vi "MasterAccelerometerSample6.vi"   [LabVIEW 2016]
uses:
  <vilib>/rvi/Emulation/niFpgaGetClockAttributes.vi
  <vilib>/rvi/Emulation/niFpgaSctlEmulationGetInTimedLoop.vi
  <vilib>/rvi/Emulation/niFpgaEmulationReportErrorSimple.vi
  <vilib>/rvi/eio/common/nirviEmuTemplateMethod_errors.vi
  <vilib>/rvi/Emulation/niFpgaEmulationIsFPGAContextNoSignature.vi
  <vilib>/rvi/DataTransferAndStorage/Container/Common/niFpgaContainerGetUniqueNameForEmu.vi
  <vilib>/rvi/Memory/Memory_Emulation/niFpgaMemoryEmulationCacheClearOnFirstRun.vi
  <vilib>/rvi/Memory/Memory_Emulation/nirvimemoryEmulationManagerCache_MakeExclusive.vi
  <vilib>/rvi/Memory/Memory_Emulation/niFpgaMemoryEmulationValidateCache.vi
  <vilib>/rvi/Memory/Memory_Emulation/nirvimemoryEmulationManagerCache_InsertValue.vi
  <vilib>/Utility/error.llb/Clear Errors.vi
  <vilib>/rvi/Memory/Memory_Emulation/nirvimemoryEmulationManagerCache_ReleaseExclusive.vi
  <vilib>/rvi/Memory/Memory_Emulation/nirvimemoryEmulationManagerCache_GetValue.vi
  <vilib>/rvi/Memory/Memory_Emulation/nirvimemoryEmulationManagerCache_SetValue.vi
  <vilib>/rvi/Emulation/niFpgaProcessEmulError.vi
  <vilib>/rvi/errors/niFpgaSetErrorForExecOnDevCompSimple.vi
  <vilib>/rvi/eio/common/nirviEmuReportErrorAndStop.vi
  <vilib>/rvi/FIFO/Fifo_Resource/nirvififoEmulationSetSize.vi
  <vilib>/rvi/FIFO/Fifo_Resource/nirviFifoEmulationQueueMgr.vi
  <instcachedir>/0/nirviFifoEmulationQueueMgr_E5CAEC123FF24DC58D834DCA3CDAA9B5.lvgen/nirviFifoEmulationQueueMgr_E5CAEC123FF24DC58D834DCA3CDAA9B5_007.vi
  <vilib>/rvi/FIFO/Fifo_Resource/nirvififoEmulationDetermineInputValidOut.vi
  <vilib>/rvi/FIFO/Fifo_Resource/nirvififoEmulationCreateLock.vi
  <vilib>/rvi/FIFO/Fifo_Resource/nirvififoEmulationObtainLock.vi
  <vilib>/rvi/FIFO/Fifo_Resource/nirvififoEmulationReleaseLock.vi
  <vilib>/rvi/occurrence/nirviWaitOnOccurrenceBase.vi
  <vilib>/rvi/errors/nirviReportUnexpectedCaseInternalError.vi
  <vilib>/rvi/errors/nirviReportUnexpectedCaseInternalError (U32).vi
  <instcachedir>/0/nirviFifoEmulationQueueMgr_E5CAEC123FF24DC58D834DCA3CDAA9B5.lvgen/nirviFifoEmulationQueueMgr_E5CAEC123FF24DC58D834DCA3CDAA9B5_005.vi
  <vilib>/rvi/Emulation/niFpgaCriticalErrorInLSC.vi
  <vilib>/eio/EIOMethodNode/EIOMethodNode.xnode
  <vilib>/eio/EIONode/EIONode.xnode
  <vilib>/rvi/DataTransferAndStorage/Container/XNode/niFpgaContainer.xnode
  <vilib>/rvi/DataTransferAndStorage/Register/Emulation/niFpgaRegisterEmulation.vi
  <vilib>/rvi/FIFO/Fifo_Resource/nirvififoEmulationWrite.vi
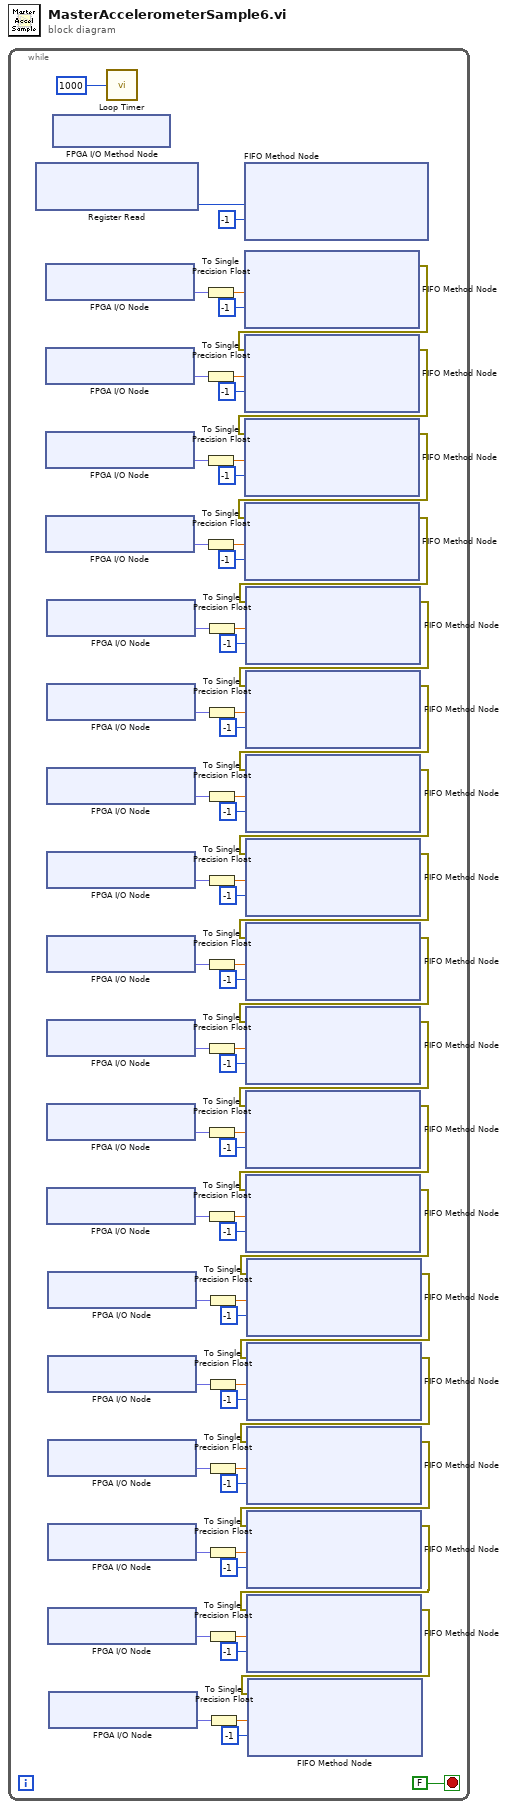
[diagram p0: block diagram]
diagram:
  n1 = while {
    stop <- FALSE stop-if-true
    n2 = xnode ("Register Read")() -> ("Data"=w60:u64)  [unwired: 1 in, 1 out]
    n3 = xnode "FPGA I/O Node"() -> ("Accelerometer1/AI0"=w72:fxp<+/-,24,7>)  [unwired: 1 in, 1 out]
    n4 = xnode "FPGA I/O Node"() -> ("Accelerometer1/AI1"=w67:fxp<+/-,24,7>)  [unwired: 1 in, 1 out]
    n5 = xnode "FPGA I/O Node"() -> ("Accelerometer1/AI2"=w62:fxp<+/-,24,7>)  [unwired: 1 in, 1 out]
    n6 = xnode "FPGA I/O Node"() -> ("Accelerometer2/AI0"=w59:fxp<+/-,24,7>)  [unwired: 1 in, 1 out]
    n7 = xnode "FPGA I/O Node"() -> ("Accelerometer2/AI1"=w42:fxp<+/-,24,7>)  [unwired: 1 in, 1 out]
    n8 = xnode "FPGA I/O Node"() -> ("Accelerometer2/AI2"=w47:fxp<+/-,24,7>)  [unwired: 1 in, 1 out]
    n9 = xnode "FPGA I/O Node"() -> ("Accelerometer3/AI0"=w55:fxp<+/-,24,7>)  [unwired: 1 in, 1 out]
    n10 = xnode "FPGA I/O Node"() -> ("Accelerometer3/AI1"=w50:fxp<+/-,24,7>)  [unwired: 1 in, 1 out]
    n11 = xnode "FPGA I/O Node"() -> ("Accelerometer3/AI2"=w10:fxp<+/-,24,7>)  [unwired: 1 in, 1 out]
    n12 = xnode "FPGA I/O Node"() -> ("Accelerometer4/AI0"=w15:fxp<+/-,24,7>)  [unwired: 1 in, 1 out]
    n13 = xnode "FPGA I/O Node"() -> ("Accelerometer4/AI1"=w23:fxp<+/-,24,7>)  [unwired: 1 in, 1 out]
    n14 = xnode "FPGA I/O Node"() -> ("Accelerometer4/AI2"=w18:fxp<+/-,24,7>)  [unwired: 1 in, 1 out]
    n15 = xnode "FPGA I/O Node"() -> ("Accelerometer5/AI0"=w39:fxp<+/-,24,7>)  [unwired: 1 in, 1 out]
    n16 = xnode "FPGA I/O Node"() -> ("Accelerometer5/AI1"=w34:fxp<+/-,24,7>)  [unwired: 1 in, 1 out]
    n17 = xnode "FPGA I/O Node"() -> ("Accelerometer5/AI2"=w26:fxp<+/-,24,7>)  [unwired: 1 in, 1 out]
    n18 = xnode "FPGA I/O Node"() -> ("Accelerometer6/AI0"=w31:fxp<+/-,24,7>)  [unwired: 1 in, 1 out]
    n19 = xnode "FPGA I/O Node"() -> ("Accelerometer6/AI1"=w8:fxp<+/-,24,7>)  [unwired: 1 in, 1 out]
    n20 = xnode "FPGA I/O Node"() -> ("Accelerometer6/AI2"=w3:fxp<+/-,24,7>)  [unwired: 1 in, 1 out]
    n21 = xnode "FPGA I/O Method Node"() -> ()  [unwired: 1 in, 1 out]
    n22 = call "Loop Timer"("Count(uSec)"=u32 1000 ("Data")) -> ()  [unwired: 1 out]
    n23 = To Single Precision Float(number=w72) -> (single precision float=w71:sgl)
    n24 = To Single Precision Float(number=w67) -> (single precision float=w68:sgl)
    n25 = To Single Precision Float(number=w62) -> (single precision float=w63:sgl)
    n26 = To Single Precision Float(number=w59) -> (single precision float=w58:sgl)
    n27 = To Single Precision Float(number=w42) -> (single precision float=w43:sgl)
    n28 = To Single Precision Float(number=w47) -> (single precision float=w46:sgl)
    n29 = To Single Precision Float(number=w55) -> (single precision float=w54:sgl)
    n30 = To Single Precision Float(number=w50) -> (single precision float=w51:sgl)
    n31 = To Single Precision Float(number=w10) -> (single precision float=w11:sgl)
    n32 = To Single Precision Float(number=w15) -> (single precision float=w14:sgl)
    n33 = To Single Precision Float(number=w23) -> (single precision float=w22:sgl)
    n34 = To Single Precision Float(number=w18) -> (single precision float=w19:sgl)
    n35 = To Single Precision Float(number=w39) -> (single precision float=w38:sgl)
    n36 = To Single Precision Float(number=w34) -> (single precision float=w35:sgl)
    n37 = To Single Precision Float(number=w26) -> (single precision float=w27:sgl)
    n38 = To Single Precision Float(number=w31) -> (single precision float=w30:sgl)
    n39 = To Single Precision Float(number=w8) -> (single precision float=w7:sgl)
    n40 = To Single Precision Float(number=w3) -> (single precision float=w4:sgl)
    n41 = xnode ("FIFO Method Node")("Element"=w60, "Timeout"=-1) -> ()  [unwired: 1 in, 2 out]
    n42 = xnode ("FIFO Method Node")("Element"=w71, "Timeout"=-1) -> ("error out"=w66:errorcluster)  [unwired: 2 in, 2 out]
    n43 = xnode ("FIFO Method Node")("Element"=w68, "Timeout"=-1, "error in (no error)"=w66) -> ("error out"=w61:errorcluster)  [unwired: 1 in, 2 out]
    n44 = xnode ("FIFO Method Node")("Element"=w63, "Timeout"=-1, "error in (no error)"=w61) -> ("error out"=w65:errorcluster)  [unwired: 1 in, 2 out]
    n45 = xnode ("FIFO Method Node")("Element"=w58, "Timeout"=-1, "error in (no error)"=w65) -> ("error out"=w41:errorcluster)  [unwired: 1 in, 2 out]
    n46 = xnode ("FIFO Method Node")("Element"=w43, "Timeout"=-1, "error in (no error)"=w41) -> ("error out"=w48:errorcluster)  [unwired: 1 in, 2 out]
    n47 = xnode ("FIFO Method Node")("Element"=w46, "Timeout"=-1, "error in (no error)"=w48) -> ("error out"=w56:errorcluster)  [unwired: 1 in, 2 out]
    n48 = xnode ("FIFO Method Node")("Element"=w54, "Timeout"=-1, "error in (no error)"=w56) -> ("error out"=w49:errorcluster)  [unwired: 1 in, 2 out]
    n49 = xnode ("FIFO Method Node")("Element"=w51, "Timeout"=-1, "error in (no error)"=w49) -> ("error out"=w9:errorcluster)  [unwired: 1 in, 2 out]
    n50 = xnode ("FIFO Method Node")("Element"=w11, "Timeout"=-1, "error in (no error)"=w9) -> ("error out"=w16:errorcluster)  [unwired: 1 in, 2 out]
    n51 = xnode ("FIFO Method Node")("Element"=w14, "Timeout"=-1, "error in (no error)"=w16) -> ("error out"=w24:errorcluster)  [unwired: 1 in, 2 out]
    n52 = xnode ("FIFO Method Node")("Element"=w22, "Timeout"=-1, "error in (no error)"=w24) -> ("error out"=w17:errorcluster)  [unwired: 1 in, 2 out]
    n53 = xnode ("FIFO Method Node")("Element"=w19, "Timeout"=-1, "error in (no error)"=w17) -> ("error out"=w40:errorcluster)  [unwired: 1 in, 2 out]
    n54 = xnode ("FIFO Method Node")("Element"=w38, "Timeout"=-1, "error in (no error)"=w40) -> ("error out"=w33:errorcluster)  [unwired: 1 in, 2 out]
    n55 = xnode ("FIFO Method Node")("Element"=w35, "Timeout"=-1, "error in (no error)"=w33) -> ("error out"=w25:errorcluster)  [unwired: 1 in, 2 out]
    n56 = xnode ("FIFO Method Node")("Element"=w27, "Timeout"=-1, "error in (no error)"=w25) -> ("error out"=w32:errorcluster)  [unwired: 1 in, 2 out]
    n57 = xnode ("FIFO Method Node")("Element"=w30, "Timeout"=-1, "error in (no error)"=w32) -> ("error out"=w1:errorcluster)  [unwired: 1 in, 2 out]
    n58 = xnode ("FIFO Method Node")("Element"=w7, "Timeout"=-1, "error in (no error)"=w1) -> ("error out"=w2:errorcluster)  [unwired: 1 in, 2 out]
    n59 = xnode ("FIFO Method Node")("Element"=w4, "Timeout"=-1, "error in (no error)"=w2) -> ()  [unwired: 1 in, 3 out]
  }
